vi "Polyphase Filter_Get Filter Factor and Mode.vi"(11 "factor in":T2={"interpolation"=1, "decimation"=1}) -> (2 "mode":T1 items=["Default"=-1, "No Rate Change"=0, "Interpolation"=1, "Decimation"=2, "Rational"=3], 3 "factor out":T2={"interpolation"=1, "decimation"=1})   [LabVIEW 2020, in "NI_AAL_Filter.lvlib"]
uses:
  <vilib>/Analysis/NI_AAL_Filter.lvlib
  <vilib>/Analysis/3filter.llb/Polyphase Filter_Factor.ctl
  <vilib>/Analysis/3filter.llb/Polyphase Filter_Mode.ctl
  <vilib>/gmath/NI_Gmath.lvlib
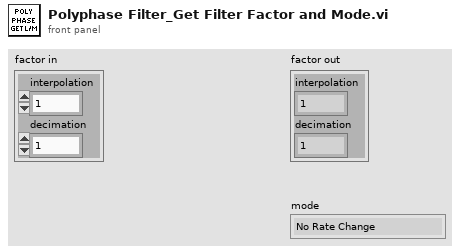
[diagram p1: front panel]
types:
  T1 = typedef "NI_AAL_Filter.lvlib/Polyphase Filter_Mode.ctl" = i32
  T2 = typedef "NI_AAL_Filter.lvlib/Polyphase Filter_Factor.ctl" = cluster{"interpolation":i32, "decimation":i32}
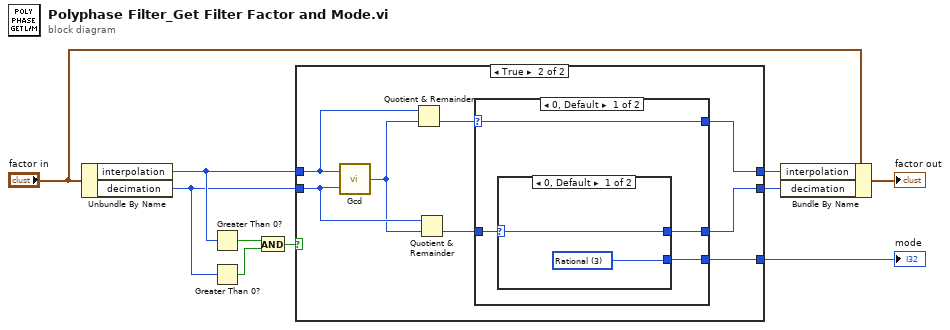
[diagram p0: block diagram]
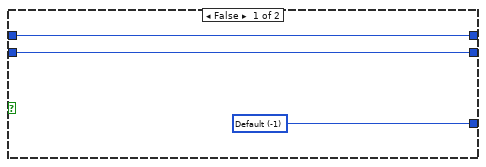
[diagram p2: hidden frame]
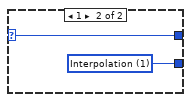
[diagram p3: hidden frame]
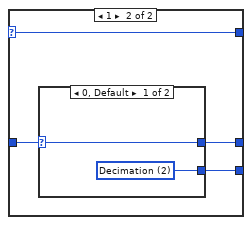
[diagram p4: hidden frame]
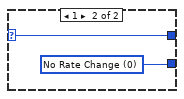
[diagram p5: hidden frame]
diagram:
  n1 = Unbundle By Name("factor in") -> ("interpolation"=w6:i32, "decimation"=w5:i32)
  n2 = Greater Than 0?(x=w6) -> (x > 0?=w3:bool)
  n3 = Greater Than 0?(x=w5) -> (x > 0?=w4:bool)
  n4 = And(x=w3, y=w4) -> (x .and. y?=w2:bool)
  n5 = case shown="True" w2 {
    tunnel: w5 -> [w12 w21]
    tunnel: w6 -> [w13 w20]
    tunnel: [w11 w18] -> w10
    tunnel: [w13 w17] -> w9
    tunnel: [w12 w16] -> w8
    frame False {
      w11 = T1 -1 items=["Default"=-1, "No Rate Change"=0, "Interpolation"=1, "Decimation"=2, "Rational"=3] ("mode")
    }
    frame True {
      n6 = call <vilib>:"Gcd.vi"("y"=w21, "x"=w20) -> ("gcd(x,y)"=w19:i32)
      n7 = Quotient & Remainder(x=w20, y=w19) -> (floor(x/y)=w15:i32)  [unwired: 1 out]
      n8 = Quotient & Remainder(x=w21, y=w19) -> (floor(x/y)=w14:i32)  [unwired: 1 out]
      n9 = case shown="0, Default" w15 {
        selector: w15 -> [w24 w32]
        tunnel: [w23 w30] -> w18
        tunnel: w14 -> [w25 w33]
        tunnel: [w24 w32] -> w17
        tunnel: [w22 w31] -> w16
        frame 0, Default {
          n10 = case shown="0, Default" w25 {
            selector: w25 -> [w27 w29]
            tunnel: [w26 w28] -> w23
            tunnel: [w27 w29] -> w22
            frame 0, Default {
              w26 = T1 3 items=["Default"=-1, "No Rate Change"=0, "Interpolation"=1, "Decimation"=2, "Rational"=3] ("mode")
            }
            frame 1 {
              w28 = T1 1 items=["Default"=-1, "No Rate Change"=0, "Interpolation"=1, "Decimation"=2, "Rational"=3] ("mode")
            }
          }
        }
        frame 1 {
          n11 = case shown="0, Default" w33 {
            selector: w33 -> [w35 w37]
            tunnel: [w35 w37] -> w31
            tunnel: [w34 w36] -> w30
            frame 0, Default {
              w34 = T1 2 items=["Default"=-1, "No Rate Change"=0, "Interpolation"=1, "Decimation"=2, "Rational"=3] ("mode")
            }
            frame 1 {
              w36 = T1 0 items=["Default"=-1, "No Rate Change"=0, "Interpolation"=1, "Decimation"=2, "Rational"=3] ("mode")
            }
          }
        }
      }
    }
  }
  "mode" <- w10
  n12 = Bundle By Name(cluster="factor in", "interpolation"=w9, "decimation"=w8) -> (→"factor out":T2)
